vi "Main Page VI Name.vi"(11 "CD Template in":refnum<class "NIVS_PPL_Inline HW Interface (Inline-Async).lvclass">) -> (2 "Main Page VI Name":string)   [LabVIEW 2019, in "NIVS_PPL_Inline HW Interface (Inline-Async).lvclass"]
uses:
  NIVS_PPL_Inline HW Interface (Inline-Async).lvclass
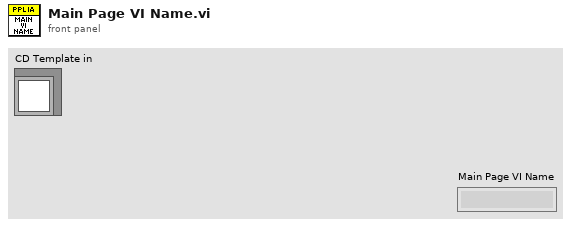
[diagram p1: front panel]
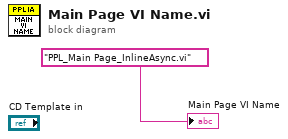
[diagram p0: block diagram]
diagram:
  "Main Page VI Name" <- "PPL_Main Page_InlineAsync.vi" ("Main Page VI Name")
